vi "Move XZ Raster  + C-Scan.vi"(0 "Reference In":refnum<class "_Controller.lvclass">, 1 "VISA resource name":refnum<visa-resource-name>, 2 "X Number of Steps":string="0", 3 "Z Number of Steps":string="0", 4 "Source (0: Channel 1)":u16(ring) items=["Channel 1", "Channel 2", "Channel 3", "Channel 4", "Memory 1", "Memory 2", "Memory 3", "Memory 4", "Function 1", "Function 2", "Function 3", "Function 4", "Function 5", "Function 6", "Function 7", "Function 8"], 5 "Error In":errorcluster, 8 "C-Scan Build Up Quantity":T1(radio), 9 "Initial X Direction":bool=TRUE, 11 "Initial Z Direction":bool=TRUE) -> (14 "Reference Out":refnum<class "_Controller.lvclass">, 16 "C-Scan":dbl[][](array[numeric]), 17 "A-Scan (for C-Scan)":waveform(dbl)[](graph), 19 "Error Out":errorcluster)   [LabVIEW 2020]
doc: "Bi-axial raster scan logic for the XZ plane inclduing the processing to obtain a C-scan from all the indiviual A-scans. Performs the uni-axial raster scan logic in the X direction then moves along 1 scanning point in the Z dirction. This is the looped to cover the entire area.\n\nArgs:\n\nReference In: Incoming communication (reference) between LabView and the scanning rig controller\nX Number of Steps: Total number of steps to move along that axis\nZ Number of Steps: Total number of steps to move along that axis\nInitial X Direction: Initial X direction for the scan\nInitial Z Direction: Initial Z direction for the scan\nC-Scan Build Up Quantity: Specifies the quantity used to build up the C-Scan image\nVISA Resource Name: Specifies the model of osciloscope being used\nSource (Channel): Specifies the channel to trigger for a reading on the osciloscope\nError In: Checks for any errors with the incoming communication (reference)\n\nReturns:\n\nReference Out: Output communnication (reference) between LabView and controller\nError Out: Checks for any error with output communication (reference)\nC-Scan: Output C-scan\nA-Scan: All the A-scan's taken for the entire plane"
uses:
  <instrlib>/Arcus Ethernet Driver 1.0.0/ArcusEthernetComm/classes/Controller/_Controller.lvclass
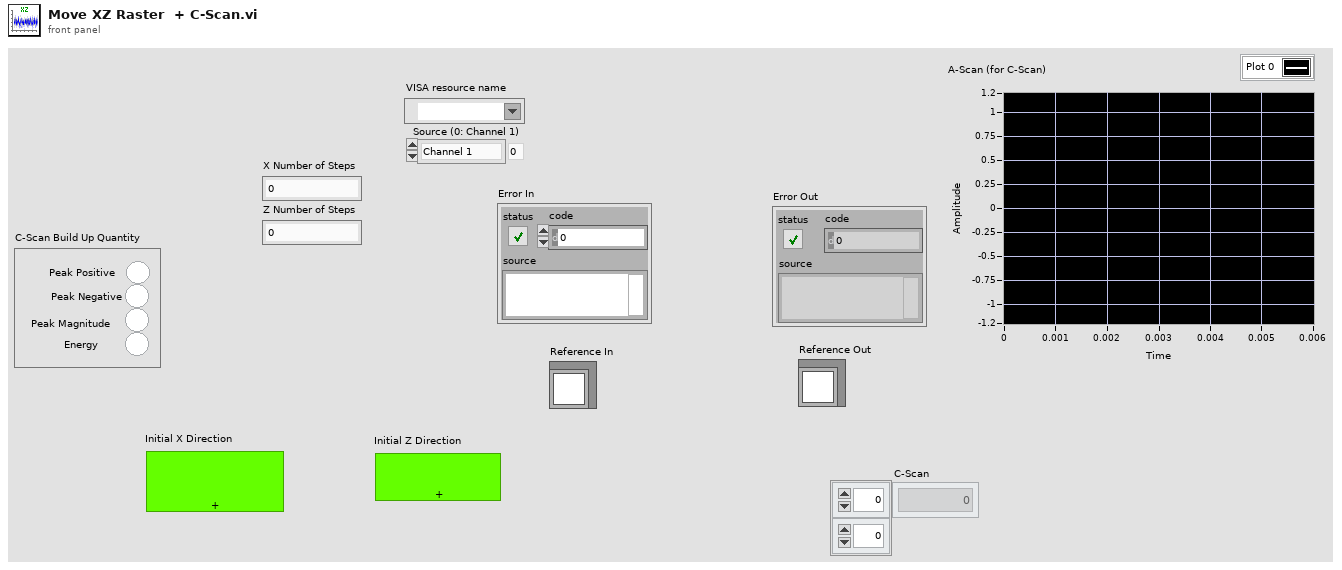
[diagram p1: front panel]
types:
  T1 = enum32{"No Selection", "Peak Positive", "Peak Negative", "Peak Magnitude", "Energy"}
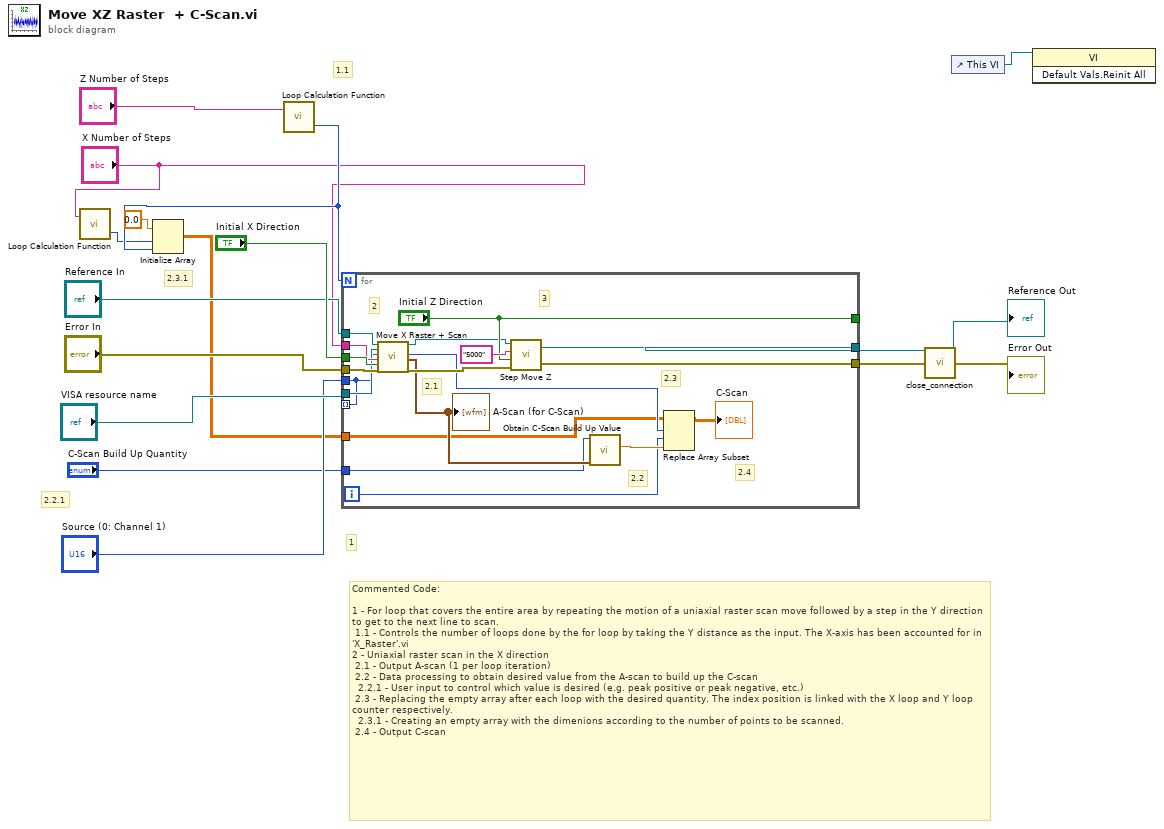
[diagram p0: block diagram]
diagram:
  # "2.3.1"
  # "2.2.1"
  # "Commented Code:\n\n1 - For loop that covers the entire area by repeating the motion of a uniaxial raster scan move followed by a step in the Y direction to get to the next line to scan.  \n 1.1 - Controls the number of loops done by the for loop by taking the Y distance as the input. The X-axis has been accounted for in 'X_Raster'.vi\n2 - Uniaxial raster scan in the X direction\n 2.1 - Output A-scan (1 per loop iteration)\n 2.2 - Data processing to obtain desired value from the A-scan to build up the C-scan\n  2.2.1 - User input to control which value is desired (e.g. peak positive or peak negative, etc.)\n 2.3 - Replacing the empty array after each loop with the desired quantity. The index position is linked with the X loop and Y loop counter respectively. \n  2.3.1 - Creating an empty array with the dimenions according to the number of points to be scanned.\n 2.4 - Output C-scan"
  # "1.1"
  # "1"
  n1 = call "Loop Calculation Function.vi"("Number of Steps"="X Number of Steps") -> ("No. of Scan Points"=w3:i32)  [unwired: 1 in, 1 out]
  n2 = call "Loop Calculation Function.vi"("Number of Steps"="Z Number of Steps") -> ("No. of Scan Points"=w4:i32)  [unwired: 1 in, 1 out]
  n3 = Initialize Array(0.0 ("element"), w3, w4) -> (w5:dbl[][])
  n4 = for {
    N: w4 -> [_]
    tunnel: "X Number of Steps" -> [w34]
    tunnel: "Initial X Direction" -> [w35]
    tunnel: ["Initial Z Direction"] -> _
    tunnel: [w31] -> w10
    tunnel: [w30] -> w9
    tunnel: "Reference In" -> [w28]
    tunnel: "Error In" -> [w27]
    tunnel: "VISA resource name" -> [w26]
    tunnel: [w25] -> _ mode=indexing
    tunnel: "Source (0: Channel 1)" -> [w25]
    tunnel: w5 -> [w20]
    tunnel: "C-Scan Build Up Quantity" -> [w18]
    i -> [w22]
    # "2.4"
    # "2.3"
    # "2.2"
    # "3"
    # "2.1"
    # "2"
    n5 = call "Move X Raster + Scan.vi"("Reference In"=w28, "VISA resource name (Osc. Model)"=w26, "Source (0: Channel 1)"=w25, "X Number of Steps"=w34, "Initial Direction"=w35, "Error In"=w27) -> ("Reference Out"=w32:refnum<class "_Controller.lvclass">, "For Loop Count"=w21:i32, "A-Scan"=w23:waveform(dbl)[], "Error Out"=w29:errorcluster)  [unwired: 10 in]
    "A-Scan (for C-Scan)" <- w23
    n6 = call "Step Move Z.vi"("Error In"=w29, "Direction"="Initial Z Direction", "No. of Z Steps"="5000" ("Y Steps"), "Reference In"=w32) -> ("Error Out"=w30:errorcluster, "Reference Out"=w31:refnum<class "_Controller.lvclass">)
    n7 = call "Obtain C-Scan Build Up Value.vi"("A-Scans"=w23, "C-Scan Build Up Quantity"=w18) -> ("Desired Value for C-Scan"=w24:dbl)  [unwired: 9 in]
    n8 = Replace Array Subset(array=w20, new element=w24, index (row)=w21, index (col)=w22) -> (→"C-Scan":dbl[][])
  }
  n9 = call <instrlib>:"close_connection.vi"("reference (in)"=w10, "error in (no error)"=w9) -> ("reference (out)"=→"Reference Out":refnum<class "_Controller.lvclass">, "error out"=→"Error Out":errorcluster)  [unwired: 16 in]
  n10 = control-ref of="This VI"() -> (w12:refnum<vi>)
  n11 = invoke class="VI" method="Default Vals.Reinit All"(reference=w12) -> ()  [unwired: 2 in, 3 out]
